vi "Get_Sweep_Start_Wavelength.vi"(8 "error in (no error)":errorcluster, 11 ".NET Reference in":refnum<k24>) -> (0 "error out":errorcluster, 2 "Start wavelength":dbl, 3 ".NET Reference out":refnum<k24>)   [LabVIEW 2017]
uses:
  D:/test/FULLband-sts/Fullband_Sample/DLL/InstrumentDLL.dll
  DLL/InstrumentDLL.dll
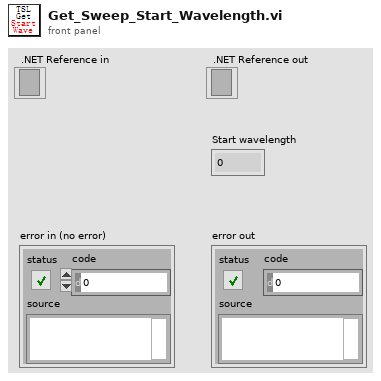
[diagram p1: front panel]
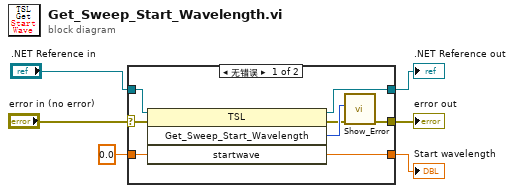
[diagram p0: block diagram]
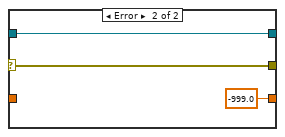
[diagram p2: hidden frame]
diagram:
  n1 = case shown="无错误" "error in (no error)" {
    selector: "error in (no error)" -> [w7 w17]
    tunnel: [w8 w17] -> w6
    tunnel: [w14 w16] -> w5
    tunnel: ".NET Reference in" -> [w13 w16]
    tunnel: [w12 -999.0 ("startwave")] -> w3
    tunnel: 0.0 ("endwave") -> [w11 _]
    frame No Error {
      n2 = invoke on="调用节点" class="TSL" method="Get_Sweep_Start_Wavelength"(reference=w13, error in=w7, "startwave"=w11) -> (reference out=w14:refnum<k24>, error out=w9:errorcluster, "Get_Sweep_Start_Wavelength"=w10:i32, "startwave"=w12:dbl)  [unwired: 1 in]
      n3 = call "Show_Error.vi"("error in (no error)"=w9, "Error"=w10) -> ("error out"=w8:errorcluster)  [unwired: 9 in]
    }
    frame Error {
    }
  }
  "Start wavelength" <- w3
  "error out" <- w6
  ".NET Reference out" <- w5
